vi "Remote Connection Manager Loop.vi"(8 "System Control":refnum<queue>, 10 "IsCloneVI (false)":bool, 11 "Remote":refnum<queue>) -> (0 "error out":errorcluster)   [LabVIEW 2020, in "SQSnobFit Control Panel.lvlib" / "Remote Connection Manager.lvlib"]
uses:
  Remote Connection Manager.lvlib
  support/Message Queue/Message Cluster.ctl
  RCM Sender Data.ctl
  <userlib>/Dynamic Reentrant/Type Defs/Message.ctl
  Instrument Manager/Instrument State.ctl
  <vilib>/addons/zeromq/zmq_context.lvclass
  <vilib>/addons/zeromq/zmq_socket.lvclass
  RCM Receiver Data.ctl
  <vilib>/ErrorRing/Error Ring.xnode
  <userlib>/Dynamic Reentrant/Dynamic Reentrant.lvlib
  support/Message Queue/Message Queue.lvlib
  Instrument Manager/Instrument Manager.lvlib
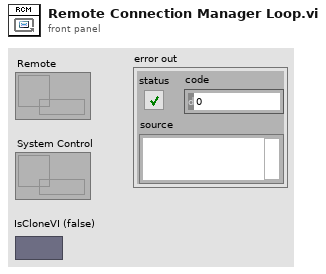
[diagram p1: front panel]
types:
  T1 = typedef "SQSnobFit Control Panel.lvlib/Remote Connection Manager.lvlib/RCM Sender Data.ctl" = cluster{"Remote VI Queue":refnum<queue>, "Remote Message List":string[]}
  T2 = typedef "Dynamic Reentrant.lvlib/Message.ctl" = cluster{"Source":string, "Destination":string, "Time Stamp":timestamp, "Command":string, "Data":variant}
  T3 = typedef "SQSnobFit Control Panel.lvlib/Instrument Manager.lvlib/Instrument State.ctl" = cluster{"Context":refnum<class "zmq_context.lvclass">, "Socket":refnum<class "zmq_socket.lvclass">, "Running Since":timestamp, "New Parameters (values)":cluster{"Time Stamp":timestamp, "Name":string[], "Value":dbl[]}, "Optimizer Path":path, "Running":bool, "Response Counter":u8, "Response Timeout (ms)":u32, "Response Retries":u32, "Endpoint":string, "Starting up?":bool, "New Parameters (percents)":cluster{"Time Stamp":timestamp, "Name":string[], "Value":dbl[]}, "Flow Rate Constant":dbl, "Yield":dbl, "Current Best (values)":cluster{"Parameter Names":string[], "Parameter Values":dbl[], "Function Value":dbl}}
  T4 = typedef "SQSnobFit Control Panel.lvlib/Remote Connection Manager.lvlib/RCM Receiver Data.ctl" = cluster{"This VI Queue":refnum<queue>}
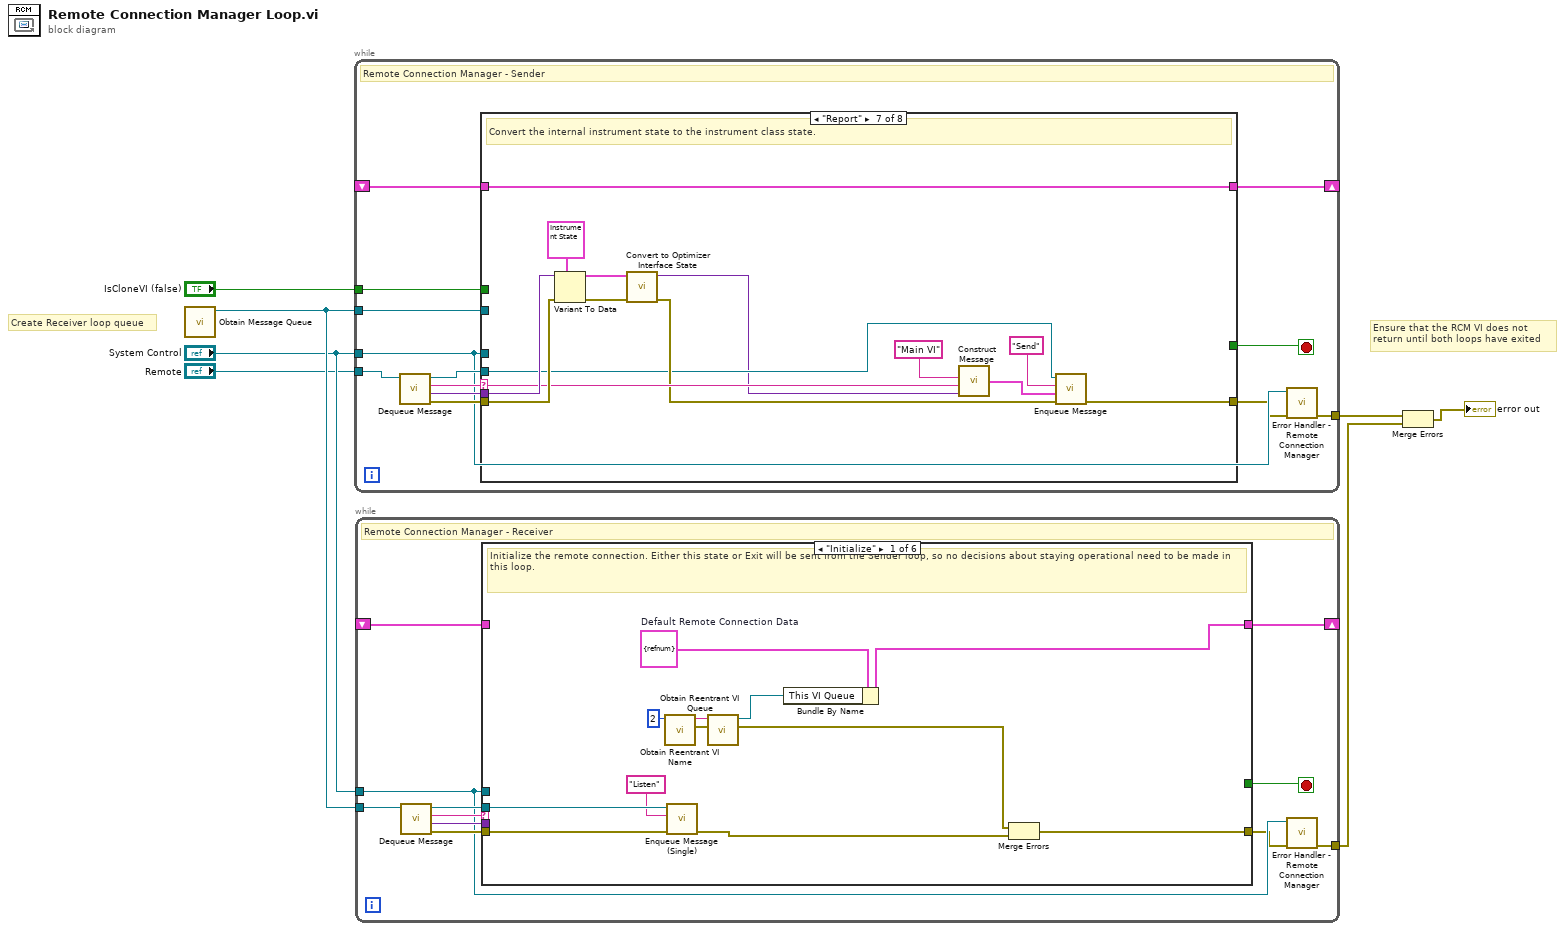
[diagram p0: block diagram]
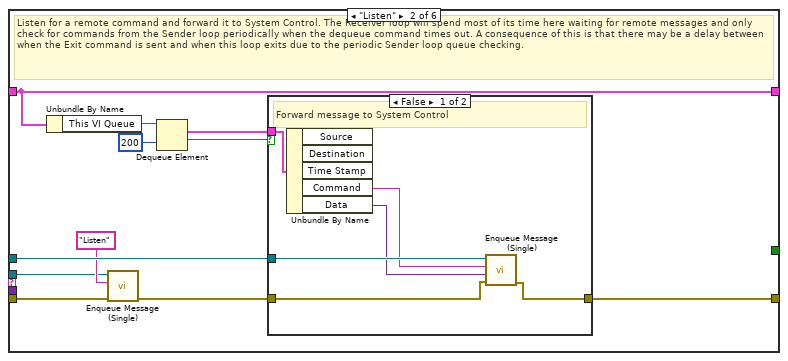
[diagram p2: hidden frame]
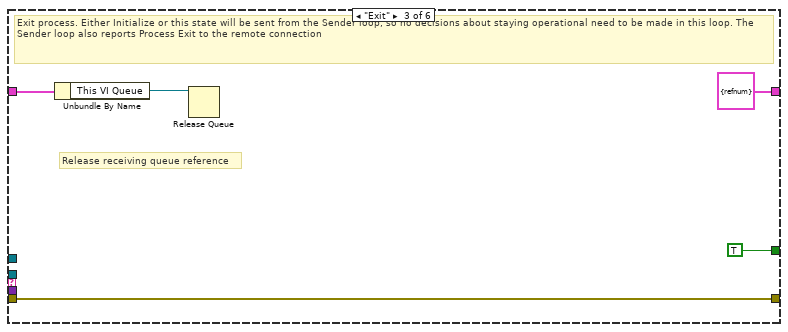
[diagram p4: hidden frame]
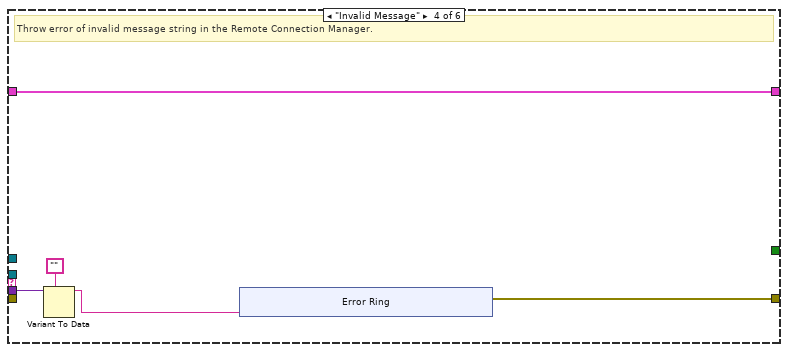
[diagram p5: hidden frame]
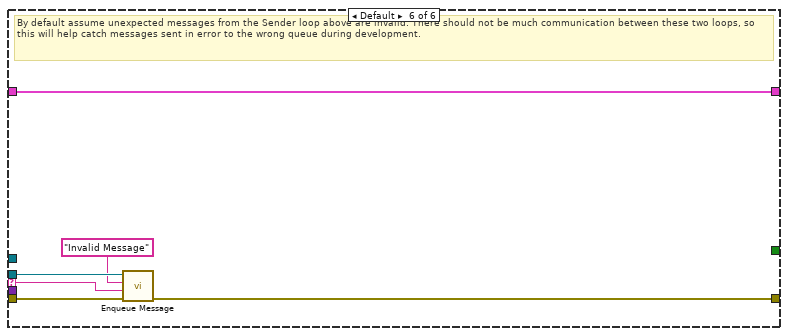
[diagram p7: hidden frame]
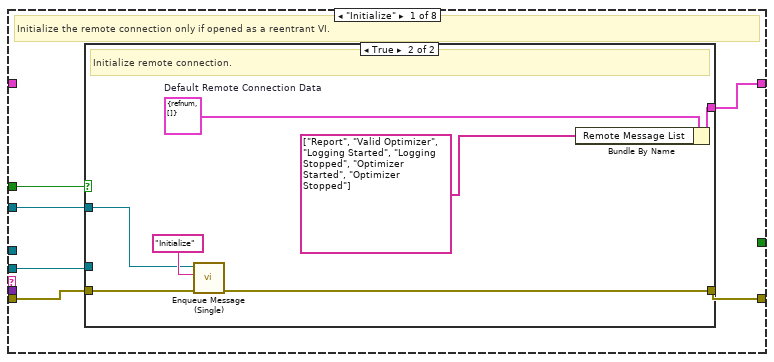
[diagram p8: hidden frame]
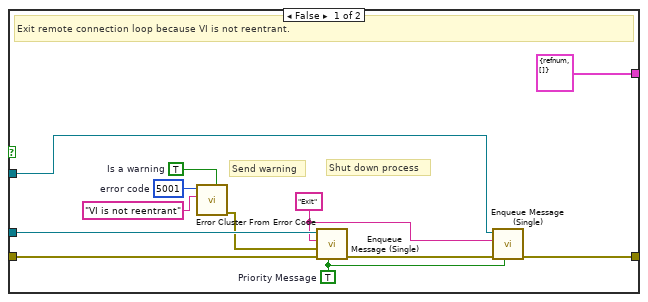
[diagram p9: hidden frame]
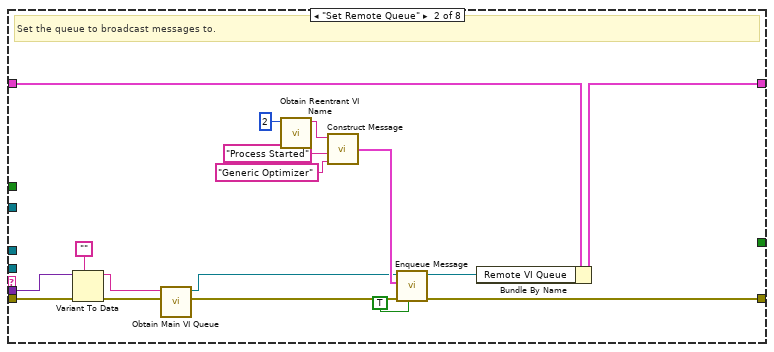
[diagram p10: hidden frame]
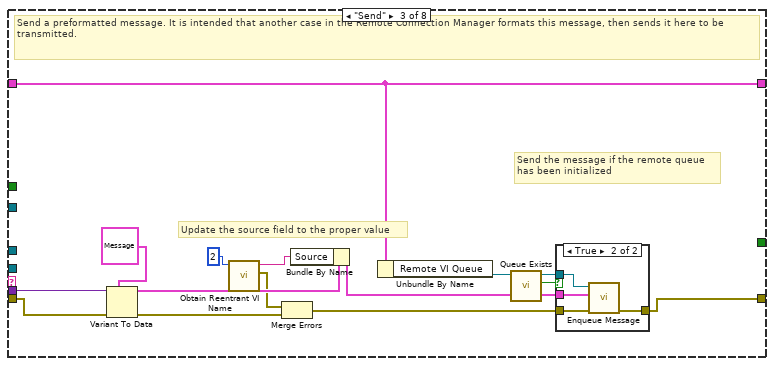
[diagram p11: hidden frame]
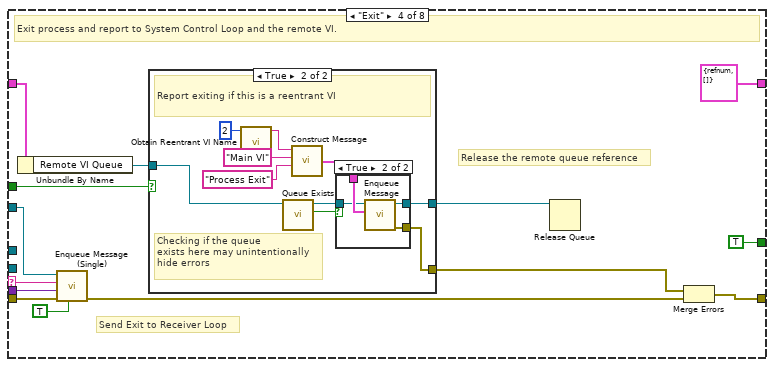
[diagram p13: hidden frame]
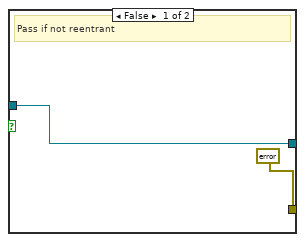
[diagram p14: hidden frame]
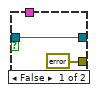
[diagram p15: hidden frame]
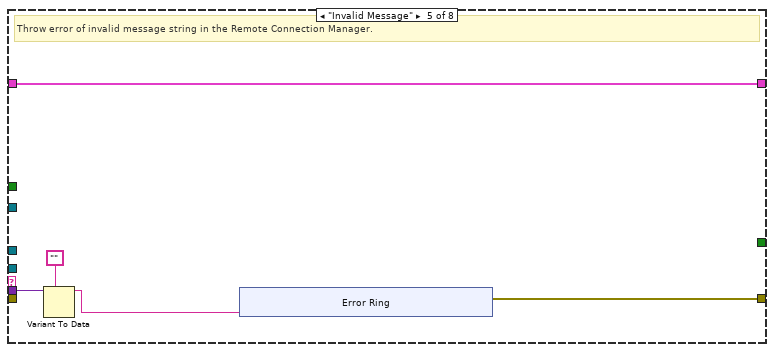
[diagram p16: hidden frame]
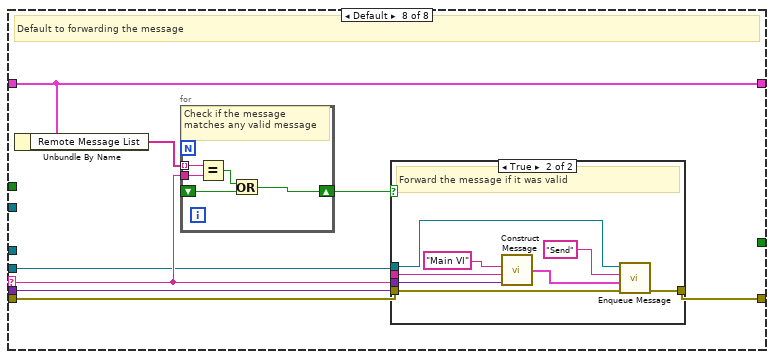
[diagram p18: hidden frame]
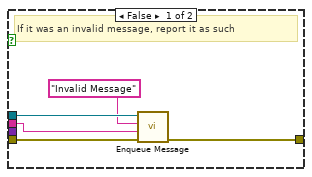
[diagram p19: hidden frame]
diagram:
  # "Create Receiver loop queue"
  # "Ensure that the RCM VI does not \nreturn until both loops have exited"
  n1 = call "Obtain Message Queue.vi"() -> ("Message Queue"=w4:refnum<queue>)  [unwired: 10 in, 1 out]
  n2 = while {
    tunnel: "Remote" -> [w19]
    tunnel: "System Control" -> [w15]
    shift-right: [w12] -> _
    shift-left: _ -> [w13]
    tunnel: [w10] -> w7
    tunnel: "IsCloneVI (false)" -> [w9]
    tunnel: w4 -> [w8]
    stop <- w11 stop-if-true
    # "Remote Connection Manager - Sender"
    n3 = call "Dequeue Message.vi"("Message Queue"=w19) -> ("error out"=w16:errorcluster, "Message Data"=w18:variant, "Message"=w20:string, "dup Message Queue"=w17:refnum<queue>)  [unwired: 7 in]
    n4 = case shown="\"Report\"" w20 {
      selector: w20 -> [_ _ _ w86 _ _ w135 w145]
      tunnel: w18 -> [_ w55 w76 w84 w117 _ w141 w146]
      tunnel: w17 -> [w25 _ _ _ _ _ w130 w144]
      tunnel: w16 -> [w24 w56 w72 w88 _ w127 w140 w147]
      tunnel: w15 -> [_ _ _ _ _ _ _ _]
      tunnel: [w23 w51 w73 w94 w119 w127 w131 w148] -> w14
      tunnel: w13 -> [_ w58 w66 w91 w118 w128 w142 w150]
      tunnel: [w26 w57 w66 T1 {"Remote VI Queue"=refnum, "Remote Message List"=[]} ("Default Remote Connection Data") w118 w128 w142 w150] -> w12
      tunnel: [_ _ _ TRUE _ _ _ _] -> w11
      tunnel: w9 -> [w22 _ _ w92 _ _ _ _]
      tunnel: w8 -> [w21 _ _ w85 _ _ _ _]
      frame "Initialize" {
        # "Initialize the remote connection only if opened as a reentrant VI."
        n5 = case shown="True" w22 {
          tunnel: [T1 {"Remote VI Queue"=refnum, "Remote Message List"=[]} ("Default Remote Connection Data") w42] -> w26
          tunnel: [w31 w43] -> w23
          tunnel: w25 -> [w34 _]
          tunnel: w24 -> [w35 w44]
          tunnel: w21 -> [w30 w41]
          frame False {
            w28 = TRUE  # Priority Message
            w29 = "Exit" ("Message")
            w36 = TRUE  # Is a warning
            w37 = 5001  # error code
            # "Shut down process"
            # "Send warning"
            # "Exit remote connection loop because VI is not reentrant."
            n6 = call <vilib>:"Error Cluster From Error Code.vi"("is warning? (False)"=w36, "error message (\"\")"="VI is not reentrant" ("error message (\"\")"), "error code (0)"=w37) -> ("error out"=w33:errorcluster)  [unwired: 6 in]
            n7 = call "Enqueue Message (Single).vi"("Priority Message? (F)"=w28, "error in (no error)"=w35, "Message Data"=w33, "Message"=w29, "Message Queue"=w34) -> ("error out"=w32:errorcluster)  [unwired: 5 in, 1 out]
            n8 = call "Enqueue Message (Single).vi"("Priority Message? (F)"=w28, "error in (no error)"=w32, "Message"=w29, "Message Queue"=w30) -> ("error out"=w31:errorcluster)  [unwired: 6 in, 1 out]
          }
          frame True {
            w40 = T1 {"Remote VI Queue"=refnum, "Remote Message List"=[]}  # Default Remote Connection Data
            # "Initialize remote connection."
            n9 = call "Enqueue Message (Single).vi"("error in (no error)"=w44, "Message"="Initialize", "Message Queue"=w41) -> ("error out"=w43:errorcluster)  [unwired: 7 in, 1 out]
            n10 = Bundle By Name(cluster=w40, "Remote Message List"=string[] ["Report", "Valid Optimizer", "Logging Started", "Logging Stopped", "Optimizer Started", "Optimizer Stopped"]) -> (w42:T1)
          }
        }
      }
      frame "Set Remote Queue" {
        # "Set the queue to broadcast messages to."
        n11 = Variant To Data(error in=w56, type="", Variant=w55) -> (data=w47:string, error out=w50:errorcluster)
        n12 = call <userlib>:"Obtain Main VI Queue.vi"("error in (no error)"=w50, "Name (Main VI)"=w47) -> ("error out"=w48:errorcluster, "queue out"=w46:refnum<queue>)  [unwired: 8 in]
        n13 = call <userlib>:"Obtain Reentrant VI Name.vi"("Call Depth (1)"=2) -> ("Clone Name"=w62:string)  [unwired: 9 in, 1 out]
        n14 = call <userlib>:"Construct Message.vi"("Data"="Generic Optimizer", "Command"="Process Started", "Source"=w62) -> ("output cluster"=w52:T2)  [unwired: 3 in]
        n15 = call <userlib>:"Enqueue Message.vi"("Priority Message? (F)"=TRUE, "error in (no error)"=w48, "Message"=w52, "Listening Queue"=w46) -> ("error out"=w51:errorcluster, "queue out"=w54:refnum<queue>)  [unwired: 6 in]
        n16 = Bundle By Name(cluster=w58, "Remote VI Queue"=w54) -> (w57:T1)
      }
      frame "Send" {
        # "Send the message if the remote queue\nhas been initialized"
        # "Update the source field to the proper value"
        # "Send a preformatted message. It is intended that another case in the Remote Connection Manager formats this message, then sends it here to be transmitted."
        n17 = Variant To Data(error in=w72, type=T2 {"Source"="", "Destination"="", "Time Stamp"=timestamp(0 s since 1904-01-01), "Command"="", "Data"=variant} ("Message"), Variant=w76) -> (data=w74:T2, error out=w75:errorcluster)
        n18 = call <userlib>:"Obtain Reentrant VI Name.vi"("Call Depth (1)"=2) -> ("error out"=w67:errorcluster, "Clone Name"=w69:string)  [unwired: 9 in]
        n19 = Merge Errors(w67, w75) -> (w68:errorcluster)
        n20 = Bundle By Name(cluster=w74, "Source"=w69) -> (w71:T2)
        n21 = Unbundle By Name(w66) -> ("Remote VI Queue"=w65:refnum<queue>)
        n22 = call <userlib>:"Queue Exists.vi"("Remote VI Queue in"=w65) -> ("Queue Exists"=w63:bool, "Remote VI Queue out"=w64:refnum<queue>)  [unwired: 9 in]
        n23 = case shown="True" w63 {
          tunnel: [w78 w82] -> w73
          tunnel: w71 -> [_ w81]
          tunnel: w68 -> [w78 w80]
          tunnel: w64 -> [_ w79]
          frame False {
          }
          frame True {
            n24 = call <userlib>:"Enqueue Message.vi"("error in (no error)"=w80, "Message"=w81, "Listening Queue"=w79) -> ("error out"=w82:errorcluster)  [unwired: 7 in, 1 out]
          }
        }
      }
      frame "Exit" {
        # "Send Exit to Receiver Loop"
        # "Release the remote queue reference"
        # "Exit process and report to System Control Loop and the remote VI."
        n25 = Unbundle By Name(w91) -> ("Remote VI Queue"=w90:refnum<queue>)
        n26 = call "Enqueue Message (Single).vi"("Priority Message? (F)"=TRUE, "error in (no error)"=w88, "Message Data"=w84, "Message"=w86, "Message Queue"=w85) -> ("error out"=w87:errorcluster)  [unwired: 5 in, 1 out]
        n27 = case shown="True" w92 {
          tunnel: [errorcluster {"status"=FALSE, "code"=0, "source"=""} ("error out") w100] -> w93
          tunnel: w90 -> [w97 w103]
          tunnel: [w97 w101] -> w89
          frame False {
            # "Pass if not reentrant"
          }
          frame True {
            # "Checking if the queue\nexists here may unintentionally\nhide errors"
            # "Report exiting if this is a reentrant VI"
            n28 = call <userlib>:"Obtain Reentrant VI Name.vi"("Call Depth (1)"=2) -> ("Clone Name"=w107:string)  [unwired: 9 in, 1 out]
            n29 = call <userlib>:"Queue Exists.vi"("Remote VI Queue in"=w103) -> ("Queue Exists"=w99:bool, "Remote VI Queue out"=w102:refnum<queue>)  [unwired: 9 in]
            n30 = call <userlib>:"Construct Message.vi"("Command"="Process Exit", "Destination"="Main VI", "Source"=w107) -> ("output cluster"=w108:T2)  [unwired: 3 in]
            n31 = case shown="True" w99 {
              tunnel: w108 -> [_ w114]
              tunnel: [w109 w113] -> w101
              tunnel: w102 -> [w109 w112]
              tunnel: [errorcluster {"status"=FALSE, "code"=0, "source"=""} ("error out") w111] -> w100
              frame False {
              }
              frame True {
                n32 = call <userlib>:"Enqueue Message.vi"("Message"=w114, "Listening Queue"=w112) -> ("error out"=w111:errorcluster, "queue out"=w113:refnum<queue>)  [unwired: 8 in]
              }
            }
          }
        }
        n33 = Release Queue(queue=w89) -> ()  [unwired: 2 in, 3 out]
        n34 = Merge Errors(w93, w87) -> (w94:errorcluster)
      }
      frame "Invalid Message" {
        # "Throw error of invalid message string in the Remote Connection Manager."
        n35 = Variant To Data(type="", Variant=w117) -> (data=w115:string)  [unwired: 1 in, 1 out]
        n36 = xnode "Error Ring"("parameter 0"=w115) -> ("error out"=w119:errorcluster)
      }
      frame "--- Copy This Frame ---" {
        # "Duplicate this frame to respond to other instrument specific messages."
      }
      frame "Report" {
        # "Convert the internal instrument state to the instrument class state."
        n37 = Variant To Data(error in=w140, type=T3 {"Context"=refnum, "Socket"=refnum, "Running Since"=timestamp(0 s since 1904-01-01), "New Parameters (values)"={"Time Stamp"=timestamp(0 s since 1904-01-01), "Name"=[], "Value"=[]}, "Optimizer Path"=path "", "Running"=FALSE, "Response Counter"=0, "Response Timeout (ms)"=0, "Response Retries"=0, "Endpoint"="", "Starting up?"=FALSE, "New Parameters (percents)"={"Time Stamp"=timestamp(0 s since 1904-01-01), "Name"=[], "Value"=[]}, "Flow Rate Constant"=0.0, "Yield"=0.0, "Current Best (values)"={"Parameter Names"=[], "Parameter Values"=[], "Function Value"=0.0}} ("Instrument State"), Variant=w141) -> (data=w137:T3, error out=w138:errorcluster)
        n38 = call "Convert to Optimizer Interface State.vi"("error in (no error)"=w138, "Optimizer State in"=w137) -> ("error out"=w134:errorcluster, "Optimizer State out"=w129:variant)  [unwired: 8 in]
        n39 = call <userlib>:"Construct Message.vi"("Data"=w129, "Command"=w135, "Destination"="Main VI") -> ("output cluster"=w132:T2)  [unwired: 3 in]
        n40 = call-poly <userlib>:"Enqueue Message.vi"("error in (no error)"=w134, "Message Data"=w132, "Message"="Send", "Message Queue"=w130) -> ("error out"=w131:errorcluster)  [unwired: 6 in, 1 out]
      }
      frame Default {
        # "Default to forwarding the message"
        n41 = Unbundle By Name(w150) -> ("Remote Message List"=w149:string[])
        n42 = for {
          tunnel: w149 -> [w167] mode=indexing
          tunnel: w145 -> [w168]
          shift-right: [w164] -> w143
          shift-left: _ -> [w165]
          # "Check if the message matches any valid message"
          n43 = Equal?(x=w167, y=w168) -> (x = y?=w166:bool)
          n44 = Or(x=w166, y=w165) -> (x .or. y?=w164:bool)
        }
        n45 = case shown="True" w143 {
          tunnel: [w154 w163] -> w148
          tunnel: w147 -> [w155 w162]
          tunnel: w146 -> [_ w160]
          tunnel: w145 -> [w153 w159]
          tunnel: w144 -> [w152 w157]
          frame False {
            # "If it was an invalid message, report it as such"
            n46 = call-poly <userlib>:"Enqueue Message.vi"("error in (no error)"=w155, "Message Data"=w153, "Message"="Invalid Message", "Message Queue"=w152) -> ("error out"=w154:errorcluster)  [unwired: 6 in, 1 out]
          }
          frame True {
            # "Forward the message if it was valid"
            n47 = call <userlib>:"Construct Message.vi"("Data"=w160, "Command"=w159, "Destination"="Main VI") -> ("output cluster"=w161:T2)  [unwired: 3 in]
            n48 = call-poly <userlib>:"Enqueue Message.vi"("error in (no error)"=w162, "Message Data"=w161, "Message"="Send", "Message Queue"=w157) -> ("error out"=w163:errorcluster)  [unwired: 6 in, 1 out]
          }
        }
      }
    }
    n49 = call "Error Handler - Remote Connection Manager.vi"("error in (no error)"=w14, "Message Queue"=w15) -> ("dup error in"=w10:errorcluster)  [unwired: 8 in, 1 out]
  }
  n50 = while {
    tunnel: w4 -> [w178]
    tunnel: "System Control" -> [w174]
    shift-right: [w171] -> _
    shift-left: _ -> [w172]
    tunnel: [w169] -> w6
    stop <- w170 stop-if-true
    # "Remote Connection Manager - Receiver"
    n51 = call "Dequeue Message.vi"("Message Queue"=w178) -> ("error out"=w175:errorcluster, "Message Data"=w177:variant, "Message"=w179:string, "dup Message Queue"=w176:refnum<queue>)  [unwired: 7 in]
    n52 = case shown="\"Initialize\"" w179 {
      selector: w179 -> [_ _ _ _ _ w231]
      tunnel: w177 -> [_ _ _ w217 _ _]
      tunnel: w176 -> [w190 w194 _ _ _ w230]
      tunnel: w175 -> [w189 w196 w214 _ w227 w232]
      tunnel: w174 -> [_ w198 _ _ _ _]
      tunnel: [w188 w192 w214 w219 w227 w233] -> w173
      tunnel: w172 -> [_ w193 w210 w218 w228 w234]
      tunnel: [w191 w193 T4 {"This VI Queue"=refnum} ("Default Remote Connection Data") w218 w228 w234] -> w171
      tunnel: [_ _ TRUE _ _ _] -> w170
      frame "Initialize" {
        w187 = T4 {"This VI Queue"=refnum}  # Default Remote Connection Data
        # "Initialize the remote connection. Either this state or Exit will be sent from the Sender loop, so no decisions about staying operational need to be made in this loop."
        n53 = call <userlib>:"Obtain Reentrant VI Name.vi"("Call Depth (1)"=2) -> ("error out"=w185:errorcluster, "Clone Name"=w184:string)  [unwired: 9 in]
        n54 = call "Enqueue Message (Single).vi"("error in (no error)"=w189, "Message"="Listen", "Message Queue"=w190) -> ("error out"=w181:errorcluster)  [unwired: 7 in, 1 out]
        n55 = call <userlib>:"Obtain Reentrant VI Queue.vi"("error in (no error)"=w185, "Name"=w184) -> ("error out"=w183:errorcluster, "queue out"=w186:refnum<queue>)  [unwired: 8 in]
        n56 = Bundle By Name(cluster=w187, "This VI Queue"=w186) -> (w191:T4)
        n57 = Merge Errors(w183, w181) -> (w188:errorcluster)
      }
      frame "Listen" {
        # "Listen for a remote command and forward it to System Control. The Receiver loop will spend most of its time here waiting for remote messages and only check for commands from the Sender loop periodically when the dequeue command times out. A consequence of this is that there may be a delay between when the Exit command is sent and when this loop exits due to the periodic Sender loop queue checking."
        n58 = Unbundle By Name(w193) -> ("This VI Queue"=w202:refnum<queue>)
        n59 = call "Enqueue Message (Single).vi"("error in (no error)"=w196, "Message"="Listen", "Message Queue"=w194) -> ("error out"=w195:errorcluster)  [unwired: 7 in, 1 out]
        n60 = Dequeue Element(queue=w202, timeout in ms (-1)=200) -> (element=w199:T2, timed out?=w200:bool)  [unwired: 1 in, 2 out]
        n61 = case shown="False" w200 {
          tunnel: w199 -> [w208 _]
          tunnel: w195 -> [w205 w209]
          tunnel: [w204 w209] -> w192
          tunnel: w198 -> [w207 _]
          frame False {
            # "Forward message to System Control"
            n62 = Unbundle By Name(w208) -> ("Command"=w203:string, "Data"=w206:variant)  [unwired: 3 out]
            n63 = call "Enqueue Message (Single).vi"("error in (no error)"=w205, "Message Data"=w206, "Message"=w203, "Message Queue"=w207) -> ("error out"=w204:errorcluster)  [unwired: 6 in, 1 out]
          }
          frame True {
            # "If timeout occurs, listen again."
          }
        }
      }
      frame "Exit" {
        # "Release receiving queue reference"
        # "Exit process. Either Initialize or this state will be sent from the Sender loop, so no decisions about staying operational need to be made in this loop. The Sender loop also reports Process Exit to the remote connection"
        n64 = Unbundle By Name(w210) -> ("This VI Queue"=w213:refnum<queue>)
        n65 = Release Queue(queue=w213) -> ()  [unwired: 2 in, 3 out]
      }
      frame "Invalid Message" {
        # "Throw error of invalid message string in the Remote Connection Manager."
        n66 = Variant To Data(type="", Variant=w217) -> (data=w215:string)  [unwired: 1 in, 1 out]
        n67 = xnode "Error Ring"("parameter 0"=w215) -> ("error out"=w219:errorcluster)
      }
      frame "--- Copy This Frame ---" {
        # "Duplicate this frame to respond to other instrument specific messages."
      }
      frame Default {
        # "By default assume unexpected messages from the Sender loop above are invalid. There should not be much communication between these two loops, so this will help catch messages sent in error to the wrong queue during development."
        n68 = call-poly <userlib>:"Enqueue Message.vi"("error in (no error)"=w232, "Message Data"=w231, "Message"="Invalid Message", "Message Queue"=w230) -> ("error out"=w233:errorcluster)  [unwired: 6 in, 1 out]
      }
    }
    n69 = call "Error Handler - Remote Connection Manager.vi"("error in (no error)"=w173, "Message Queue"=w174) -> ("dup error in"=w169:errorcluster)  [unwired: 8 in, 1 out]
  }
  n70 = Merge Errors(w7, w6) -> (→"error out":errorcluster)
